vi "Copy Builds To NIVS Dir.vi"(5 "Files Generated by Build":path[](array[path]), 6 "Top Level/Always Included VIs":path[](array[path]), 7 "Destination Path":path, 8 "error in (no error)":errorcluster, 9 "Target Name":string, 10 "Build Specification Name":string, 11 "Project Path":path) -> (0 "error out":errorcluster)   [LabVIEW 2011]
uses:
  <vilib>/Utility/sysdir.llb/System Directory Type.ctl
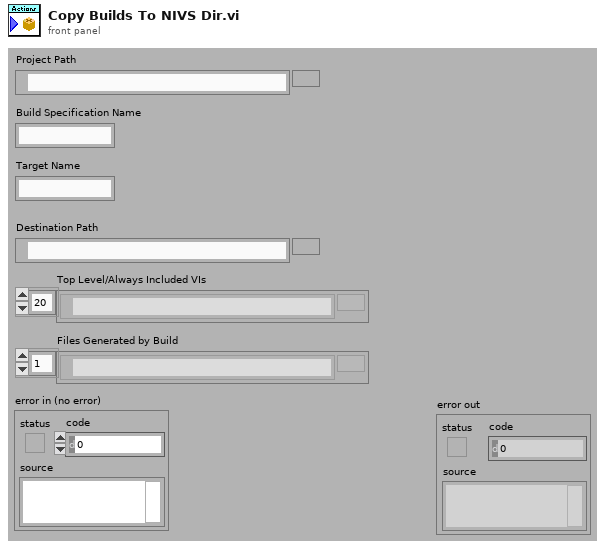
[diagram p1: front panel]
types:
  T1 = typedef "System Directory Type.ctl" = i32
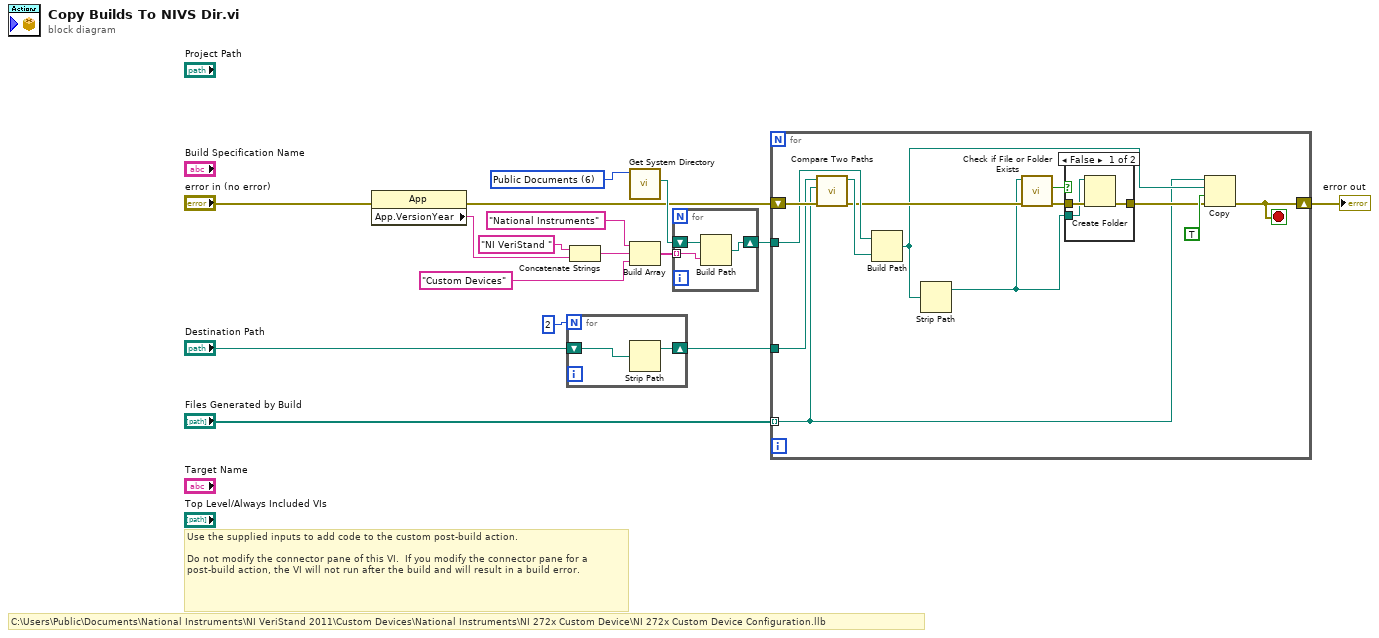
[diagram p0: block diagram]
diagram:
  w16 = T1 6 items=["User Home"=0, "User Desktop"=1, "User Documents"=2, "User Application Data"=3, "User Preferences"=4, "User Temporary"=5, "Public Documents"=6, "Public Application Data"=7, "Public Preferences"=8, "Public Cache"=13, "System Core Libraries"=9, "System Installed Libraries"=10, "Application Files"=11, "Boot Volume Root"=12] ("system directory type")
  # "C:\\Users\\Public\\Documents\\National Instruments\\NI VeriStand 2011\\Custom Devices\\National Instruments\\NI 272x Custom Device\\NI 272x Custom Device Configuration.llb"
  # "Use the supplied inputs to add code to the custom post-build action.\n\nDo not modify the connector pane of this VI.  If you modify the connector pane for a post-build action, the VI will not run after the build and will result in a build error."
  n1 = property class="App"(error in="error in (no error)") -> (error out=w6:errorcluster, "App.VersionYear"=w12:string)  [unwired: 1 in, 1 out]
  n2 = for {
    N: 2 -> [_]
    shift-right: [w17] -> w4
    shift-left: "Destination Path" -> [w18]
    n3 = Strip Path(path=w18) -> (stripped path=w17:path)  [unwired: 1 out]
  }
  n4 = Concatenate Strings("NI VeriStand " ("name or relative path"), w12) -> (w10:string)
  n5 = call <vilib>:"Get System Directory.vi"("system directory type"=w16) -> ("system directory"=w15:path)  [unwired: 10 in]
  n6 = Build Array("National Instruments" ("name or relative path"), w10, "Custom Devices" ("name or relative path")) -> (w9:string[])
  n7 = for {
    shift-right: [w20] -> w3
    shift-left: w15 -> [w21]
    tunnel: w9 -> [w19] mode=indexing
    n8 = Build Path(base path=w21, name or relative path=w19) -> (appended path=w20:path)
  }
  n9 = for {
    shift-right: [w29] -> w8
    shift-left: w6 -> [w33]
    tunnel: "Files Generated by Build" -> [w23] mode=indexing
    tunnel: w3 -> [w32]
    tunnel: w4 -> [w30]
    stop <- w29 stop-if-true
    n10 = call <vilib>:"Compare Two Paths.vi"("error in (no error)"=w33, "Path 2"=w23, "Path 1"=w30) -> ("error out"=w28:errorcluster, "Relative Path from 1 to 2"=w31:path)  [unwired: 5 in, 2 out]
    n11 = Build Path(base path=w32, name or relative path=w31) -> (appended path=w24:path)
    n12 = Strip Path(path=w24) -> (stripped path=w22:path)  [unwired: 1 out]
    n13 = call <vilib>:"Check if File or Folder Exists.vi"("error in (no error)"=w28, "path"=w22) -> ("error out"=w26:errorcluster, "file or folder exists?"=w27:bool)  [unwired: 7 in, 1 out]
    n14 = case shown="False" w27 {
      tunnel: w26 -> [w37 w38]
      tunnel: [w36 w38] -> w25
      tunnel: w22 -> [w35 _]
      frame False {
        n15 = Create Folder(path (use dialog)=w35, error in=w37) -> (error out=w36:errorcluster)  [unwired: 1 in, 2 out]
      }
      frame True {
      }
    }
    n16 = Copy(8:w25, 9:TRUE ("overwrite (F)"), 10:w24, 11:w23) -> (0:w29:errorcluster)  [unwired: 1 in, 2 out]
  }
  "error out" <- w8
